vi "x(t)积分.vi"() -> ()   [LabVIEW 2018]
uses:
  <vilib>/Analysis/2dsp.llb/Integral Method.ctl
  <vilib>/Analysis/NI_AALPro.lvlib
panel:
  in  "integration method":T1=1 caption="积分方法" items=["梯形法则", "Simpson法则", "Simpson 3/8法则", "Bode法则"]
  out "结果":dbl[](array[numeric])
  in  "数组":dbl[](array[numeric])
  in  "dt":dbl=1.0
  in  "Final Condition":dbl[](array[numeric])=[0.0] caption="最终条件"
  in  "Initial Condition":dbl[](array[numeric])=[0.0] caption="初始条件"
  in  "停止":bool
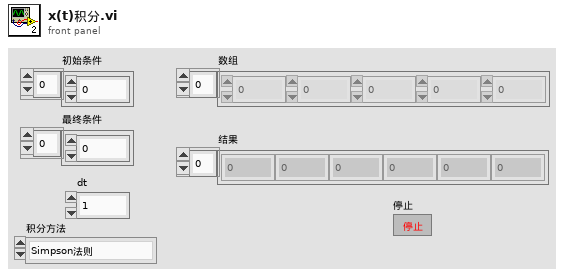
[diagram p1: front panel]
types:
  T1 = typedef "NI_AALPro.lvlib/Integral Method.ctl" = i32
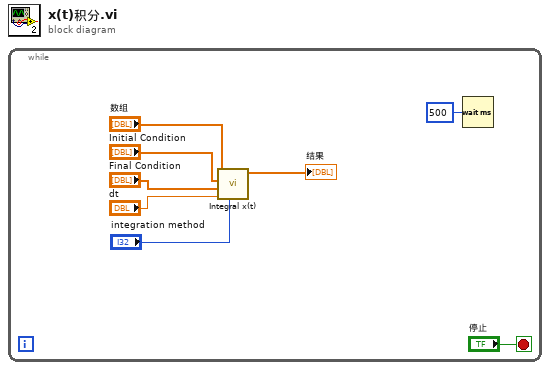
[diagram p0: block diagram]
diagram:
  n1 = while {
    stop <- "停止" stop-if-true
    n2 = call <vilib>:"Integral x(t).vi"("integration method"="integration method", "dt"="dt", "Final Condition"="Final Condition", "Initial Condition"="Initial Condition", "X"="数组") -> ("Integral X"=→"结果":dbl[])  [unwired: 5 in, 1 out]
    n3 = Wait (ms)(milliseconds to wait=u32 500 ("等待时间（毫秒）")) -> ()  [unwired: 1 out]
  }
